vi "SIM Init From Cluster (user cluster).vi"(4 "errorin":errorcluster, 6 "Sim Params":T1={"Initial Time"=0.0, "Final Time"=10.0, "Time Step"=0.1, "Absolute Tolerance"=0.001, "Relative Tolerance"=1e-06, "Continuous Solver"=enum."Adams-Moulton (variable)", "Discrete Time Step"=2.0, "Minimum Time Step"=1e-06, "Maximum Time Step"=0.1, "Initial Time Step"=0.01} {"Initial Time Step" min=0.0; "Maximum Time Step" min=0.0}) -> (1 "Simulation data out":T3={"continuous integrator"=enum."RK 1 (Euler)", "initial time"=0.0, "final time"=0.0, "step size"=0.0, "proposed step size"=0.0, "max step size"=0.0, "min step size"=0.0, "discrete time step"=0.0, "max step ratio"=0.0, "Diag Eval Stage"=enum."Init", "Substep Index"=0, "Timestep Index"=0.0, "simulation time"=0.0, "current timestep base"=0.0, "proposed step time"=0.0, "absolute tolerance"=0.0, "relative tolerance"=0.0, "step accepted?"=FALSE, "step complete?"=FALSE, "Halt?"=FALSE, "reset integrator?"=FALSE, "machine epsilon"=0.0, "min float"=0.0, "error"={"status"=FALSE, "code"=0, "source"=""}, "Method Order"=0, "Finished Late [i-1]"=FALSE, "Discrete step?"=FALSE, "NaN and Inf check?"=FALSE, "Final Timestep Index"=0.0, "(maj+disc)or(init)?"=FALSE, "Full Solver Reset"=TRUE, "Execution Mode"=enum."Simulate to Completion", "check vector sizes?"=FALSE, "solver handles zc?"=FALSE, "Simulation Registry"={"Current Idx"=0, "Node Tags"=[], "Node Headers"=[], "Node Data"=[], "Cont State data"={"inputs"=[], "outputs"=[], "reset"=[], "lower limits"=[], "upper limits"=[], "limit types"=[], "reset types"=[], "initial conditions"=[], "reset I.C."=[], "limited?"=[], "State Names"=[]}, "DiscreteInfo"={"tick period (sec)"=0.0, "time (ticks)"=0, "fire?"=[], "registry"={"period (sec)"=[], "skew (sec)"=[], "period (tick)"=[], "skew (tick)"=[]}, "discrete \nblocks?"=FALSE, "steps per tick"=0.0, "steps to tick"=0.0, "discrete \ntick?"=FALSE}, "Disc State data"={"Disc States"=[], "State Names"=[]}, "Registry Error"={"Error Block ID"=0, "code"=0}, "ZC Indices"=[]}, "variable step solver?"=FALSE, "First Substep?"=FALSE, "Continuous States?"=FALSE} {"min float" format="%.1e"; "proposed step size" format="%.1e"; "proposed step time" format="%.1e"; "max step ratio" format="%.1e"; "min step size" format="%.1e"; "machine epsilon" format="%.1e"; "discrete time step" format="%.1e"; "max step size" format="%.1e"; "current timestep base" format="%.1e"; "final time" format="%.1e"; "simulation time" format="%.1e"; "relative tolerance" format="%.1e"; "absolute tolerance" format="%.1e"; "Substep Index" format="%.1e"; "step size" format="%.1e"; "initial time" format="%.1e"})   [LabVIEW 2020]
uses:
  <vilib>/Simulation/Implementation/Shared/SIM simulation data.ctl
  <vilib>/Simulation/Implementation/Shared/SIM integration method.ctl
  <vilib>/Simulation/Implementation/Shared/SIM diagram eval stage.ctl
  <vilib>/Simulation/Implementation/Shared/SIMSCR Execution Mode.ctl
  <vilib>/Simulation/Implementation/Shared/SIM Registry.llb/SIM Simulation Registry.ctl
  <vilib>/Simulation/Implementation/Shared/SIM Registry.llb/SIM Registry Node Header.ctl
  <vilib>/Simulation/Implementation/Shared/SIM Registry.llb/SIM Registry Node Record.ctl
  <vilib>/Simulation/Implementation/Shared/SIM trigger type.ctl
  <vilib>/Simulation/Implementation/Shared/SIM solver state data.ctl
  <vilib>/Simulation/Implementation/Shared/SIM limit type.ctl
  <vilib>/Simulation/Implementation/Shared/SIM discrete data.ctl
  <vilib>/Simulation/Implementation/Shared/SIM Discrete state data.ctl
  <vilib>/Simulation/Implementation/Shared/SIM Registry.llb/SIM Simulation Registry Error.ctl
  <vilib>/Simulation/Utility/Implementation/Shared/SIM Diagram Parameters.ctl
  <vilib>/Simulation/Implementation/Shared/SIM Continuous Solvers.ctl
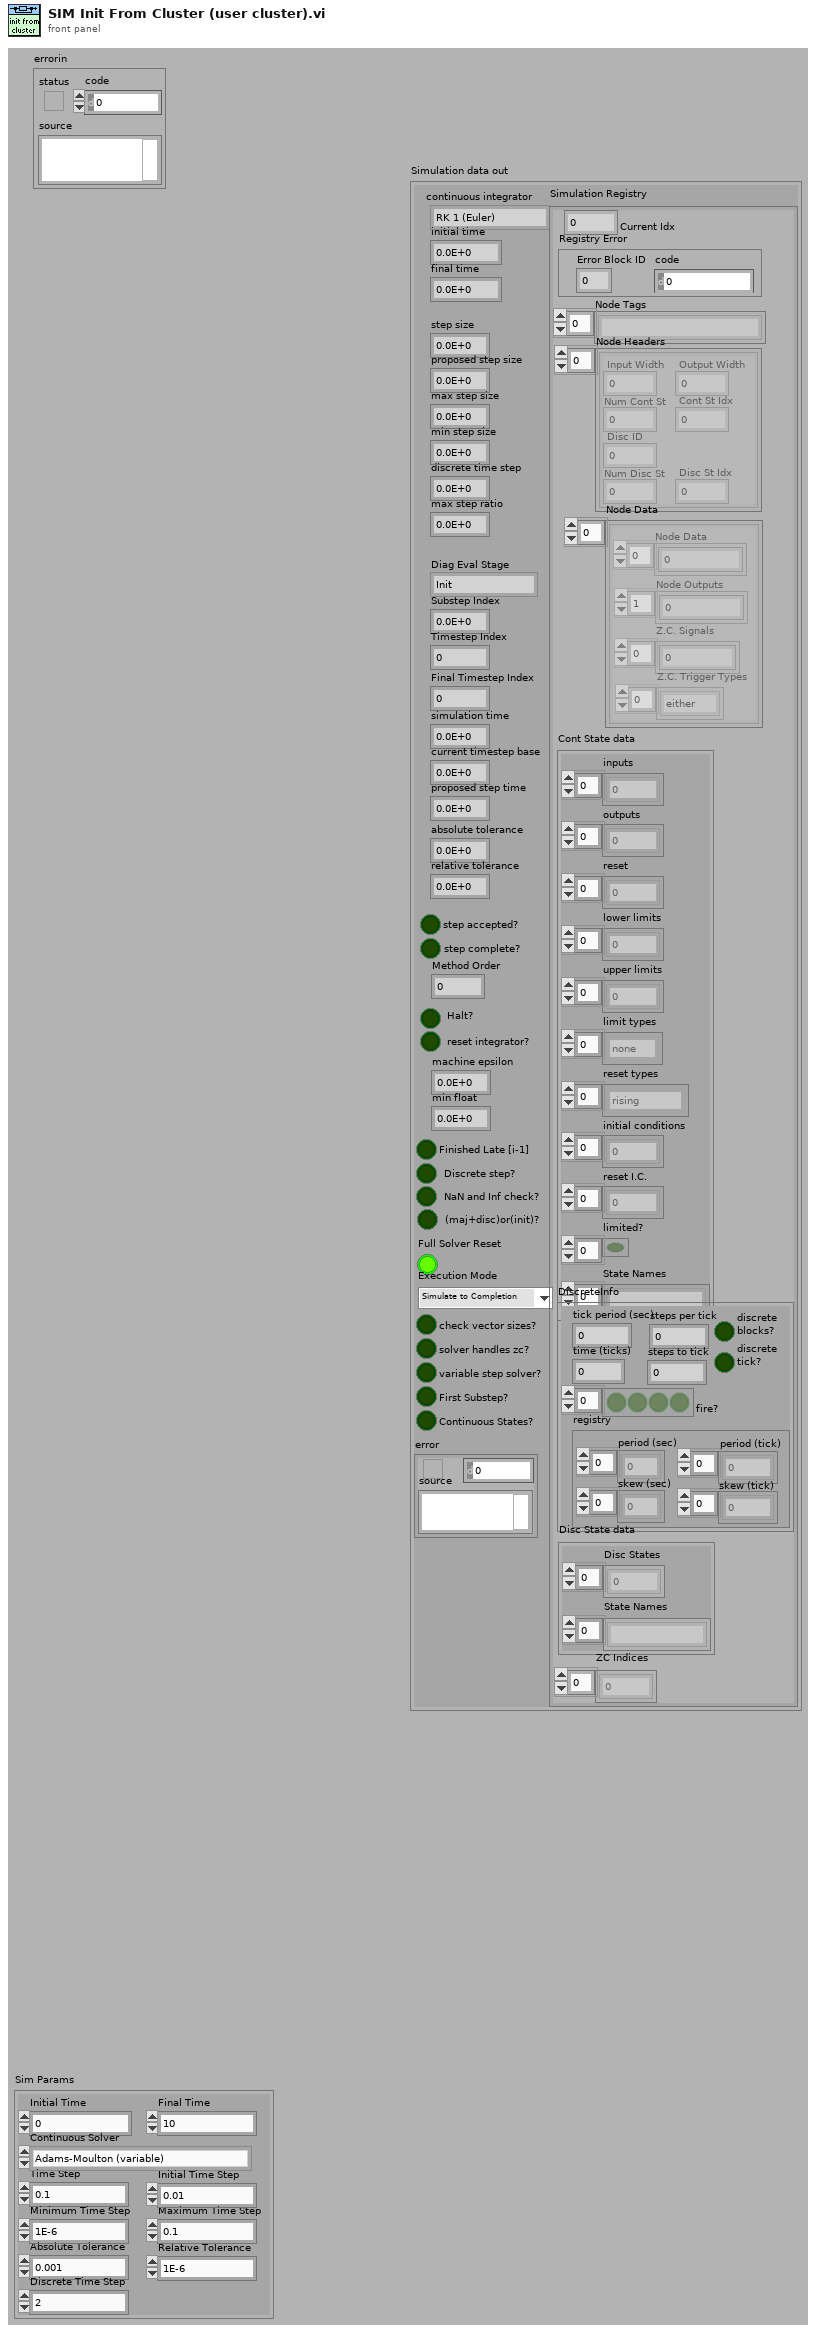
[diagram p1: front panel]
types:
  T1 = typedef "SIM Diagram Parameters.ctl" = cluster{"Initial Time":dbl, "Final Time":dbl, "Time Step":dbl, "Absolute Tolerance":dbl, "Relative Tolerance":dbl, "Continuous Solver":T2, "Discrete Time Step":dbl, "Minimum Time Step":dbl, "Maximum Time Step":dbl, "Initial Time Step":dbl}
  T2 = typedef "SIM Continuous Solvers.ctl" = enum16{"Runge-Kutta 1 (Euler)", "Runge-Kutta 2", "Runge-Kutta 3", "Runge-Kutta 4", "Runge-Kutta 23 (variable)", "Runge-Kutta 45 (variable)", "BDF (variable)", "Adams-Moulton (variable)", "Rosenbrock (variable)", "Discrete States Only"}
  T3 = typedef "SIM simulation data.ctl" = cluster{"continuous integrator":T4, "initial time":dbl, "final time":dbl, "step size":dbl, "proposed step size":dbl, "max step size":dbl, "min step size":dbl, "discrete time step":dbl, "max step ratio":dbl, "Diag Eval Stage":T5, "Substep Index":i32, "Timestep Index":dbl, "simulation time":dbl, "current timestep base":dbl, "proposed step time":dbl, "absolute tolerance":dbl, "relative tolerance":dbl, "step accepted?":bool, "step complete?":bool, "Halt?":bool, "reset integrator?":bool, "machine epsilon":dbl, "min float":dbl, "error":errorcluster, "Method Order":u32, "Finished Late [i-1]":bool, "Discrete step?":bool, "NaN and Inf check?":bool, "Final Timestep Index":dbl, "(maj+disc)or(init)?":bool, "Full Solver Reset":bool, "Execution Mode":T6, "check vector sizes?":bool, "solver handles zc?":bool, "Simulation Registry":T7, "variable step solver?":bool, "First Substep?":bool, "Continuous States?":bool}
  T4 = typedef "SIM integration method.ctl" = enum16{"RK 1 (Euler)", "Linearizer", "State Query", "Trim Eval", "Adams", "RK 3", "RK 4", "RK 45", "BDF", "RK 2", "RK 23", "Rosenbrock", "Discrete States Only"}
  T5 = typedef "SIM diagram eval stage.ctl" = enum16{"Init", "Minor Substep", "Major Substep", "Final"}
  T6 = typedef "SIMSCR Execution Mode.ctl" = enum16{"Simulate to Completion", "Single Time-Step Simulation (Fixed Step Only)"}
  T7 = typedef "SIM Simulation Registry.ctl" = cluster{"Current Idx":i32, "Node Tags":string[], "Node Headers":T8[], "Node Data":T9[], "Cont State data":T11, "DiscreteInfo":T13, "Disc State data":T14, "Registry Error":T15, "ZC Indices":i32[]}
  T8 = typedef "SIM Registry Node Header.ctl" = cluster{"Input Width":i32, "Disc ID":i32, "Num Cont St":i32, "Cont St Idx":i32, "Num Disc St":i32, "Disc St Idx":i32, "Output Width":i32}
  T9 = typedef "SIM Registry Node Record.ctl" = cluster{"Node Data":dbl[], "Node Outputs":dbl[], "Z.C. Signals":dbl[], "Z.C. Trigger Types":T10[]}
  T10 = typedef "SIM trigger type.ctl" = enum16{"rising", "falling", "either", "none"}
  T11 = typedef "SIM solver state data.ctl" = cluster{"inputs":dbl[], "outputs":dbl[], "reset":dbl[], "lower limits":dbl[], "upper limits":dbl[], "limit types":T12[], "reset types":T10[], "initial conditions":dbl[], "reset I.C.":dbl[], "limited?":bool[], "State Names":string[]}
  T12 = typedef "SIM limit type.ctl" = enum16{"upper", "lower", "both", "none"}
  T13 = typedef "SIM discrete data.ctl" = cluster{"tick period (sec)":dbl, "time (ticks)":i32, "fire?":bool[], "registry":cluster{"period (sec)":dbl[], "skew (sec)":dbl[], "period (tick)":i32[], "skew (tick)":i32[]}, "discrete \nblocks?":bool, "steps per tick":dbl, "steps to tick":dbl, "discrete \ntick?":bool}
  T14 = typedef "SIM Discrete state data.ctl" = cluster{"Disc States":dbl[], "State Names":string[]}
  T15 = typedef "SIM Simulation Registry Error.ctl" = cluster{"Error Block ID":i32, "code":i32}
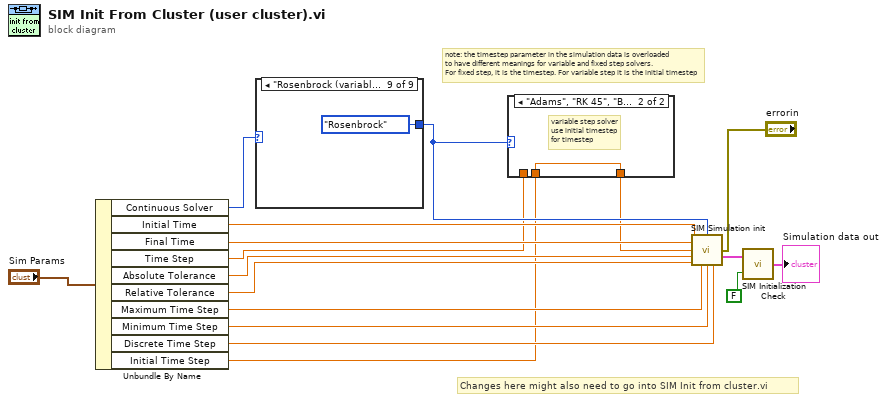
[diagram p0: block diagram]
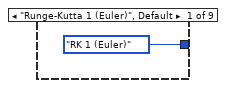
[diagram p3: hidden frame]
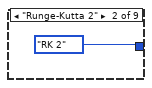
[diagram p4: hidden frame]
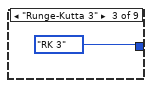
[diagram p5: hidden frame]
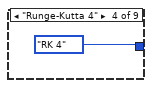
[diagram p6: hidden frame]
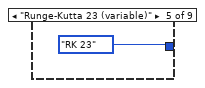
[diagram p7: hidden frame]
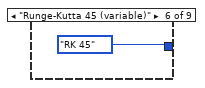
[diagram p8: hidden frame]
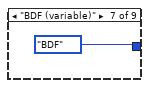
[diagram p9: hidden frame]
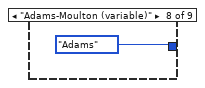
[diagram p10: hidden frame]
diagram:
  # "Changes here might also need to go into SIM Init from cluster.vi"
  # "note: the timestep parameter in the simulation data is overloaded\nto have different meanings for variable and fixed step solvers.\nFor fixed step, it is the timestep. For variable step it is the initial timestep"
  n1 = Unbundle By Name("Sim Params") -> ("Continuous Solver"=w7:T2, "Initial Time"=w14:dbl, "Final Time"=w13:dbl, "Time Step"=w3:dbl, "Absolute Tolerance"=w12:dbl, "Relative Tolerance"=w11:dbl, "Maximum Time Step"=w10:dbl, "Minimum Time Step"=w9:dbl, "Discrete Time Step"=w8:dbl, "Initial Time Step"=w2:dbl)
  n2 = case shown="\"Rosenbrock (variable)\"" w7 {
    tunnel: [SIM_integration_method."RK 1 (Euler)" ("continuous integrator") SIM_integration_method."RK 2" ("continuous integrator") SIM_integration_method."RK 3" ("continuous integrator") SIM_integration_method."RK 4" ("continuous integrator") SIM_integration_method."RK 23" ("continuous integrator") SIM_integration_method."RK 45" ("continuous integrator") SIM_integration_method."BDF" ("continuous integrator") SIM_integration_method."Adams" ("continuous integrator") SIM_integration_method."Rosenbrock" ("continuous integrator")] -> w4
    frame "Runge-Kutta 1 (Euler)", Default {
    }
    frame "Runge-Kutta 2" {
    }
    frame "Runge-Kutta 3" {
    }
    frame "Runge-Kutta 4" {
    }
    frame "Runge-Kutta 23 (variable)" {
    }
    frame "Runge-Kutta 45 (variable)" {
    }
    frame "BDF (variable)" {
    }
    frame "Adams-Moulton (variable)" {
    }
    frame "Rosenbrock (variable)" {
    }
  }
  n3 = case shown="\"Adams\", \"RK 45\", \"BDF\", \"RK 23\", \"Rosenbrock\"" w4 {
    tunnel: w3 -> [w27 _]
    tunnel: w2 -> [_ w28]
    tunnel: [w27 w28] -> w1
    frame "RK 1 (Euler)", Default {
      # "fixed step solver\nuse timestep timestep\nfor timestep"
    }
    frame "Adams", "RK 45", "BDF", "RK 23", "Rosenbrock" {
      # "variable step solver\nuse initial timestep\nfor timestep"
    }
  }
  n4 = call <vilib>:"SIM Simulation init.vi"("initial time"=w14, "continuous integrator"=w4, "final time"=w13, "time step"=w1, "error in (no error)"="errorin", "absolute tolerance"=w12, "relative tolerance"=w11, "maximum step size"=w10, "min step size"=w9, "discrete time step"=w8) -> ("Simulation data out"=w16:T3)  [unwired: 5 in]
  n5 = call <vilib>:"SIM Initialization Check.vi"("Automatic Discrete Step Size?"=FALSE, "Simulation data"=w16) -> ("Simulation data out"=→"Simulation data out":T3)
